vi "PlotHelper.vi"(5 "Y-Axis":T4, 7 "X-Axis":T4, 9 "Data_IN":T1={"Value"=0.0, "GUI Data Cluster"={"S11"=FALSE, "S21"=FALSE, "S12"=FALSE, "S22"=FALSE, "S11Meas"=enum."Log-magnitude (dB)", "S21Meas"=enum."Log-magnitude (dB)", "S12Meas"=enum."Log-magnitude (dB)", "S22Meas"=enum."Log-magnitude (dB)"}, "Timing"={"Last Operation"=0.0, "Stop @ T"=FALSE, "Delta T Log"=FALSE, "End T"=0.0, "Delta T"=0.0, "Last Temp"=0.0}, "Measurements"=[], "Hardware"={"VNA TCP Con"=refnum, "VNA TCP Port"=5025, "Global T VAR"="", "Global B VAR"=""}, "Operation"={"Operation Mode"=enum."Logging", "Status"="", "NewLog?"=FALSE}}) -> (0 "Progress Plots":cluster{"Variant X":dbl, "Variant Y":dbl}[](array[cluster]), 1 "Data_Out":T1={"Value"=0.0, "GUI Data Cluster"={"S11"=FALSE, "S21"=FALSE, "S12"=FALSE, "S22"=FALSE, "S11Meas"=enum."Log-magnitude (dB)", "S21Meas"=enum."Log-magnitude (dB)", "S12Meas"=enum."Log-magnitude (dB)", "S22Meas"=enum."Log-magnitude (dB)"}, "Timing"={"Last Operation"=0.0, "Stop @ T"=FALSE, "Delta T Log"=FALSE, "End T"=0.0, "Delta T"=0.0, "Last Temp"=0.0}, "Measurements"=[], "Hardware"={"VNA TCP Con"=refnum, "VNA TCP Port"=5025, "Global T VAR"="", "Global B VAR"=""}, "Operation"={"Operation Mode"=enum."Logging", "Status"="", "NewLog?"=FALSE}})   [LabVIEW 2021]
uses:
  Plotting-Axis.ctl
  Data_Cluster.ctl
  Measurement_Cluster.ctl
  Mode_Enum.ctl
  82b2c7e2-1130-4631-9edb-692d0da541f7.vi
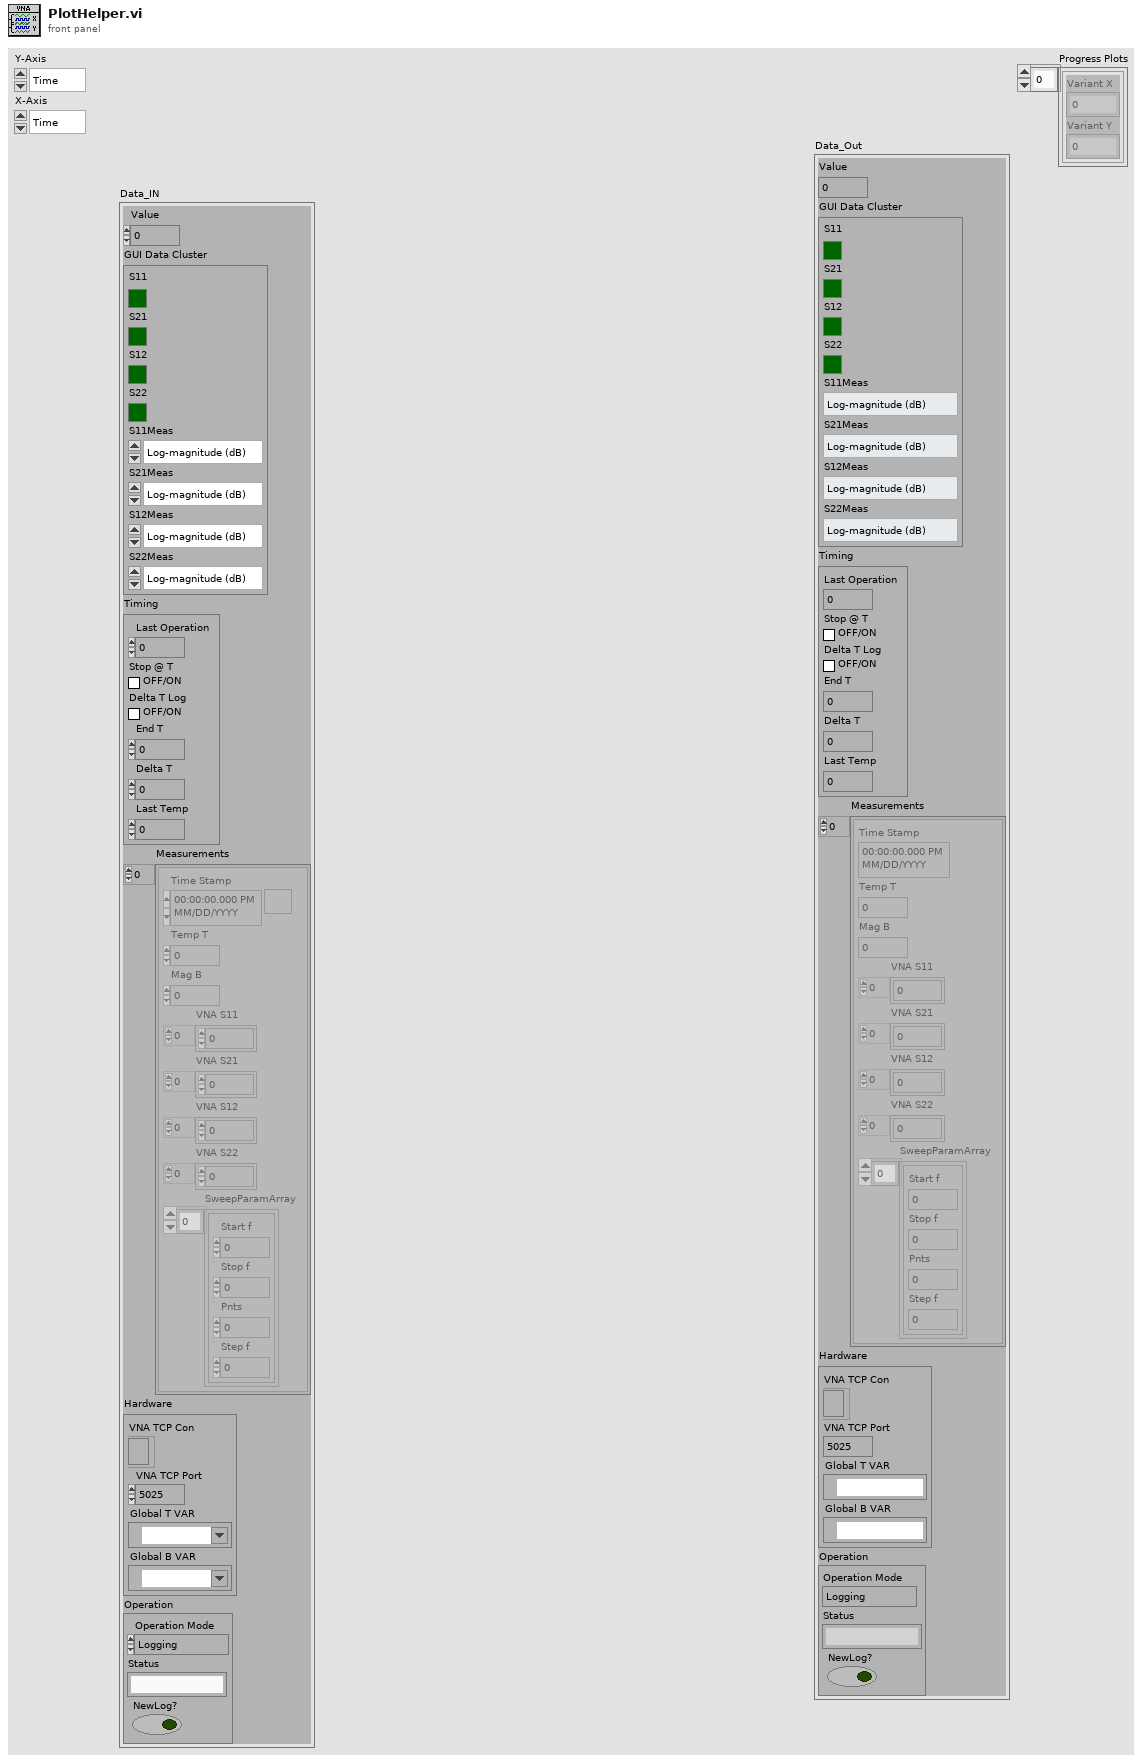
[diagram p1: front panel]
types:
  T1 = typedef "Data_Cluster.ctl" = cluster{"Value":dbl, "GUI Data Cluster":cluster{"S11":bool, "S21":bool, "S12":bool, "S22":bool, "S11Meas":enum16{"Log-magnitude (dB)", "Linear magnitude", "Phase (deg)", "Time Domain", "Real", "Imaginary", "Group Delay", "Polarlinear"}, "S21Meas":enum16{"Log-magnitude (dB)", "Linear magnitude", "Phase (deg)", "Time Domain", "Real", "Imaginary", "Group Delay", "Polarlinear"}, "S12Meas":enum16{"Log-magnitude (dB)", "Linear magnitude", "Phase (deg)", "Time Domain", "Real", "Imaginary", "Group Delay", "Polarlinear"}, "S22Meas":enum16{"Log-magnitude (dB)", "Linear magnitude", "Phase (deg)", "Time Domain", "Real", "Imaginary", "Group Delay", "Polarlinear"}}, "Timing":cluster{"Last Operation":dbl, "Stop @ T":bool, "Delta T Log":bool, "End T":dbl, "Delta T":dbl, "Last Temp":dbl}, "Measurements":T2[], "Hardware":cluster{"VNA TCP Con":refnum<k5>, "VNA TCP Port":i32, "Global T VAR":refnum<k21>, "Global B VAR":refnum<k21>}, "Operation":cluster{"Operation Mode":T3, "Status":string, "NewLog?":bool}}
  T2 = typedef "Measurement_Cluster.ctl" = cluster{"Time Stamp":timestamp, "Temp T":dbl, "Mag B":dbl, "VNA S11":dbl[], "VNA S21":dbl[], "VNA S12":dbl[], "VNA S22":dbl[], "SweepParamArray":cluster{"Start f":dbl, "Stop f":dbl, "Pnts":i32, "Step f":dbl}[]}
  T3 = typedef "Mode_Enum.ctl" = enum16{"OvenNRDY", "Logging", "Idle-Off", "Idle"}
  T4 = typedef "Plotting-Axis.ctl" = enum16{"Time", "Temperature", "Magnetic Field"}
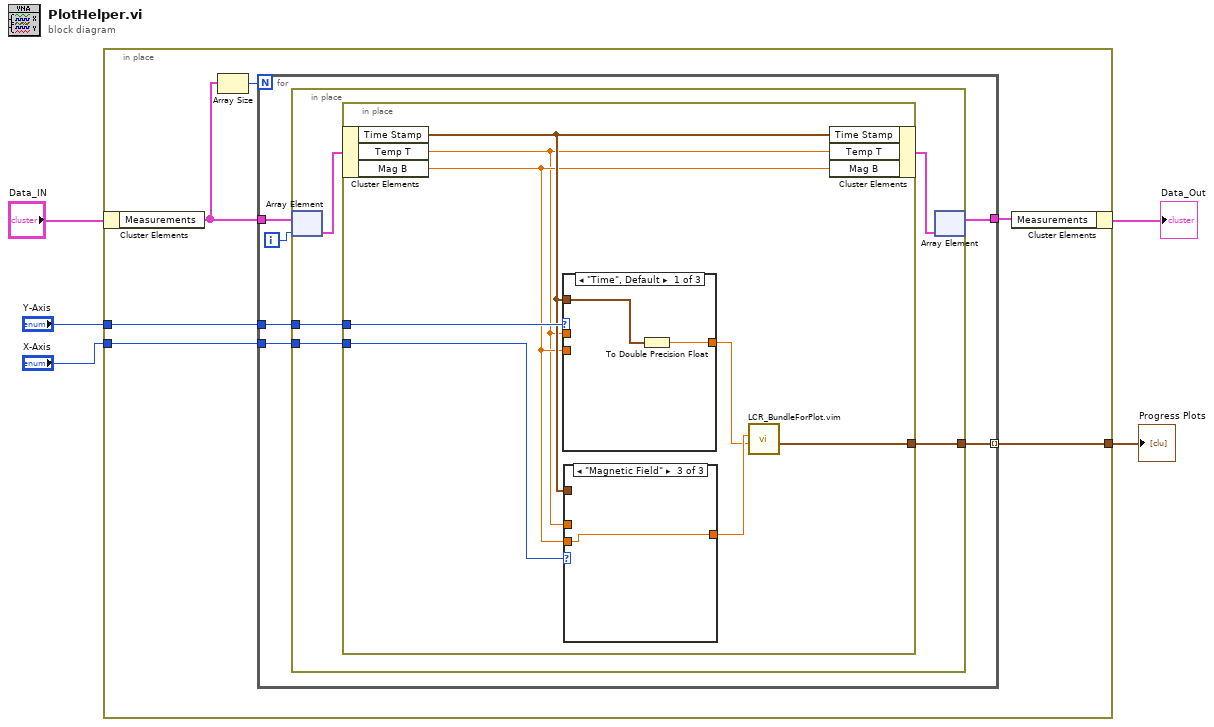
[diagram p0: block diagram]
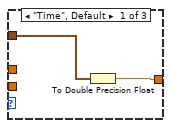
[diagram p2: hidden frame]
diagram:
  n1 = in-place {
    in-place-border: "Y-Axis" -> [w9]
    in-place-border: "X-Axis" -> [w8]
    in-place-border: [w6] -> w1
    n2 = in-place-cluster #1("Data_IN") -> ("Measurements"=w11:T2[])
    n3 = Array Size(array=w11) -> (size(s)=w10:i32)
    n4 = for {
      N: w10 -> [_]
      tunnel: w11 -> [w17]
      tunnel: w9 -> [w15]
      tunnel: w8 -> [w14]
      tunnel: [w13] -> w7
      tunnel: [w12] -> w6 mode=indexing
      i -> [w16]
      n5 = in-place {
        in-place-border: w15 -> [w21]
        in-place-border: w14 -> [w20]
        in-place-border: [w18] -> w12
        n6 = in-place-array #2(w17, w16) -> (w22:T2)
        n7 = in-place {
          in-place-border: w21 -> [w30]
          in-place-border: w20 -> [w29]
          in-place-border: [w25] -> w18
          n8 = in-place-cluster #3(w22) -> ("Time Stamp"=w27:timestamp, "Temp T"=w23:dbl, "Mag B"=w26:dbl)
          n9 = case shown="\"Time\", Default" w30 {
            tunnel: w27 -> [w36 _ _]
            tunnel: w23 -> [_ w37 _]
            tunnel: w26 -> [_ _ w38]
            tunnel: [w35 w37 w38] -> w24
            frame "Time", Default {
              n10 = To Double Precision Float(number=w36) -> (double precision float=w35:dbl)
            }
            frame "Temperature" {
            }
            frame "Magnetic Field" {
            }
          }
          n11 = case shown="\"Magnetic Field\"" w29 {
            tunnel: w27 -> [w32 _ _]
            tunnel: w23 -> [_ w33 _]
            tunnel: w26 -> [_ _ w34]
            tunnel: [w31 w33 w34] -> w28
            frame "Time", Default {
              n12 = To Double Precision Float(number=w32) -> (double precision float=w31:dbl)
            }
            frame "Temperature" {
            }
            frame "Magnetic Field" {
            }
          }
          n13 = call "LCR_BundleForPlot.vim"("Variant Y"=w24, "Variant X"=w28) -> ("Bundled Variant"=w25:cluster{"Variant X":dbl, "Variant Y":dbl})  [unwired: 9 in]
          n14 = in-place-cluster #3("Time Stamp"=w27, "Temp T"=w23, "Mag B"=w26) -> (w19:T2)
        }
        n15 = in-place-array #2(w19) -> (w13:T2[])  [unwired: 1 out]
      }
    }
    n16 = in-place-cluster #1("Measurements"=w7) -> (→"Data_Out":T1)
  }
  "Progress Plots" <- w1
